vi "Measurements Scan.vi"(8 "error in (no error)":errorcluster, 11 "Controller in":refnum<class "Controller.lvclass">) -> (0 "error out":errorcluster, 3 "Controller out":refnum<class "Controller.lvclass">)   [LabVIEW 2015, in "Controller Actor.lvlib" / "Controller.lvclass"]
uses:
  Controller.lvclass
  Controller.lvclass/Controller.ctl
  Accessors/Read Root Path.vi
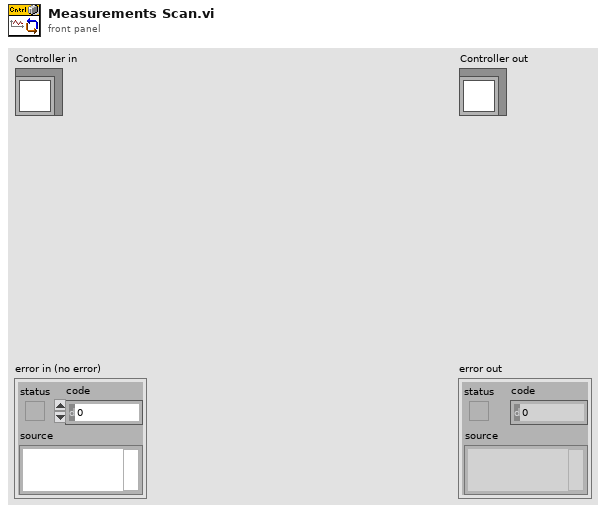
[diagram p1: front panel]
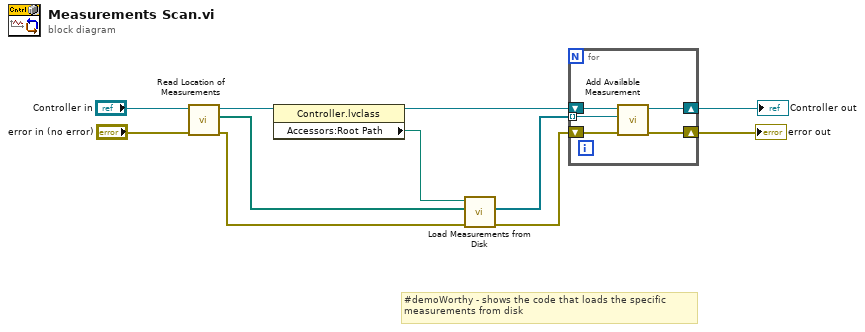
[diagram p0: block diagram]
diagram:
  # "#demoWorthy - shows the code that loads the specific\nmeasurements from disk"
  n1 = call "Read Location of Measurements.vi"("error in (no error)"="error in (no error)", "Controller in"="Controller in") -> ("error out"=w7:errorcluster, "Array of Measurement Location"=w6:path[], "Controller out"=w3:refnum<class "Controller.lvclass">)  [unwired: 7 in]
  n2 = property class="Controller.lvclass"(reference=w3) -> (reference out=w1:refnum<class "Controller.lvclass">, "Accessors:Root Path"=w2:path)  [unwired: 1 in, 1 out]
  n3 = call "Load Measurements from Disk.vi"("error in (no error)"=w7, "Array of paths (folders to scan or explicit files)"=w6, "base path"=w2) -> ("error out"=w4:errorcluster, "Available Measurements"=w5:refnum<class "Measurement.lvclass">[])  [unwired: 7 in]
  n4 = for {
    tunnel: w5 -> [w14] mode=indexing
    shift-right: [w15] -> w10
    shift-left: w1 -> [w16]
    shift-right: [w12] -> w11
    shift-left: w4 -> [w13]
    n5 = call "Add Available Measurement.vi"("error in (no error)"=w13, "Measurement.lvclass"=w14, "Controller in"=w16) -> ("error out"=w12:errorcluster, "Controller out"=w15:refnum<class "Controller.lvclass">)  [unwired: 7 in]
  }
  "error out" <- w11
  "Controller out" <- w10
